vi "DMM6500_Check_Loop_Error_FGV.vi"(5 "VI_name":string, 7 "Case":string, 8 "error in (no error)":errorcluster, 9 "queue In":refnum<queue>, 10 "Ignore Errors":i32[](array[numeric]), 11 "Exit on Error? (F)":bool) -> (3 "Boolean":bool)   [LabVIEW 2024, in "DMM6500.lvlib"]
doc: "ThisVI\n---------------------------------------------------\nCheck Loop Error List\n---------------------------------------------------\n-Checks the Error Code .\n-Eneque the \"Exit\" or \"Error\" message if error code in Ignore Error List."
uses:
  DMM6500.lvlib
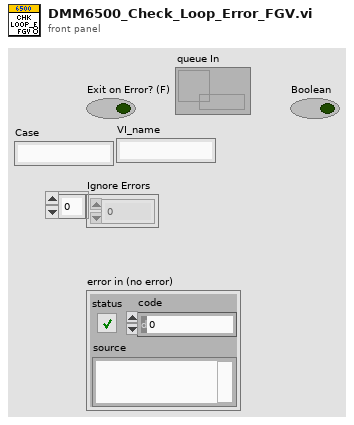
[diagram p1: front panel]
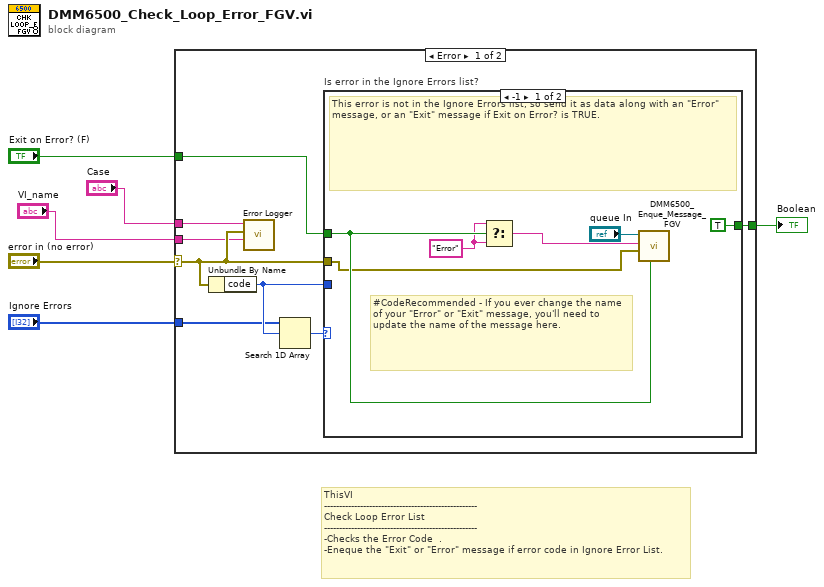
[diagram p0: block diagram]
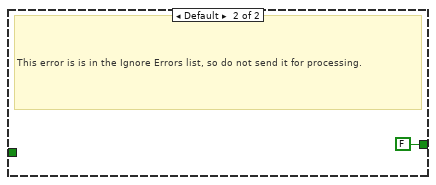
[diagram p2: hidden frame]
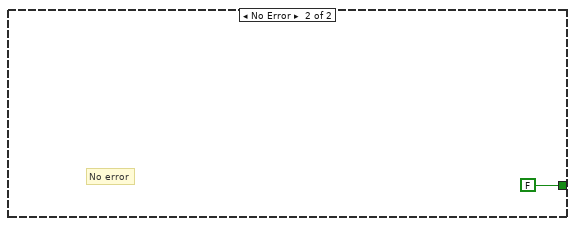
[diagram p3: hidden frame]
diagram:
  # "ThisVI\n---------------------------------------------------\nCheck Loop Error List\n---------------------------------------------------\n-Checks the Error Code  .\n-Eneque the \"Exit\" or \"Error\" message if error code in Ignore Error List."
  n1 = case shown="Error" "error in (no error)" {
    selector: "error in (no error)" -> [w8 _]
    tunnel: "Ignore Errors" -> [w12 _]
    tunnel: [w11 FALSE] -> w5
    tunnel: "Exit on Error? (F)" -> [w10 _]
    tunnel: "Case" -> [w9 _]
    tunnel: "VI_name" -> [w7 _]
    frame Error {
      n2 = Unbundle By Name(w8) -> ("code"=w13:i32)
      n3 = call "Error Logger.vi"("VI_name"=w7, "Error"=w8, "Case"=w9) -> ()  [unwired: 8 in, 1 out]
      n4 = Search 1D Array(1D array=w12, element=w13) -> (index of element=w14:i32)  [unwired: 1 in]
      n5 = case "Is error in the Ignore Errors list?" shown="-1" w14 {
        tunnel: w8 -> [w18 _]
        tunnel: w13 -> [_ _]
        tunnel: [TRUE FALSE] -> w11
        tunnel: w10 -> [w19 _]
        frame -1 {
          w16 = "Error" ("Message")
          # "#CodeRecommended - If you ever change the name of your \"Error\" or \"Exit\" message, you'll need to update the name of the message here."
          # "This error is not in the Ignore Errors list, so send it as data along with an \"Error\" message, or an \"Exit\" message if Exit on Error? is TRUE."
          n6 = Select(t=w16, s=w19, f=w16) -> (s? t:f=w17:string)
          n7 = call "DMM6500_Enque_Message_FGV.vi"("Priority"=w19, "Message Data"=w18, "Message"=w17, "queue In"="queue In") -> ()  [unwired: 7 in, 1 out]
        }
        frame Default {
          # "This error is is in the Ignore Errors list, so do not send it for processing."
        }
      }
    }
    frame No Error {
      # "No error"
    }
  }
  "Boolean" <- w5
